vi "Tag Single Channel.vi"(0 "Data in":i16[](array[numeric])=[0, 0, 0, 0], 1 "Tag Record":bool, 2 "TagData":T1, 3 "Input Valid":bool, 4 "Tag Identifier (I16)":i16=-32768, 5 "Channel":T2(ring)) -> (7 "Single Channel Data out":i16, 8 "Output Valid":bool, 9 "Pixel Overwritten by Tag":bool)   [LabVIEW 2014]
uses:
  Frametag Data.ctl
panel:
  # "Copyright 2014 Vidrio Technologies\nScanImage 5 software is licensed under the Apache License, Version 2.0 (the \"License\"); you may not use any files contained\nwithin the ScanImage 5 release except in compliance with the License. You may obtain a copy of the License at\n http://www.apache.org/licenses/LICENSE-2.0\nUnless required by applicable law or agreed to in writing, software distributed under the License is distributed on an\n\"AS IS\" BASIS, WITHOUT WARRANTIES OR CONDITIONS OF ANY KIND, either express or implied. See the License for the\n specific language governing permissions and limitations under the License."
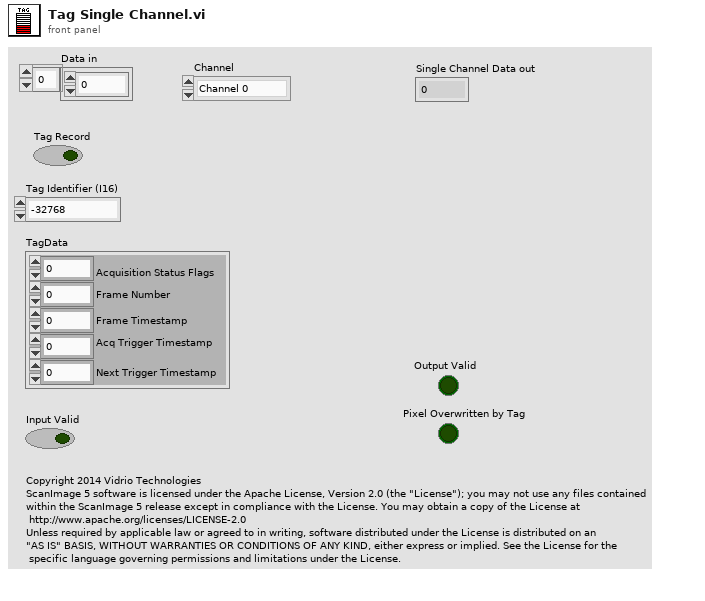
[diagram p1: front panel]
types:
  T1 = typedef "Frametag Data.ctl" = cluster{"Acquisition Status Flags":u16, "Frame Number":u32, "Frame Timestamp":u64, "Acq Trigger Timestamp":u64, "Next Trigger Timestamp":u64}
  T2 = enum8{"Channel 0", "Channel 1", "Channel 2", "Channel 3"}
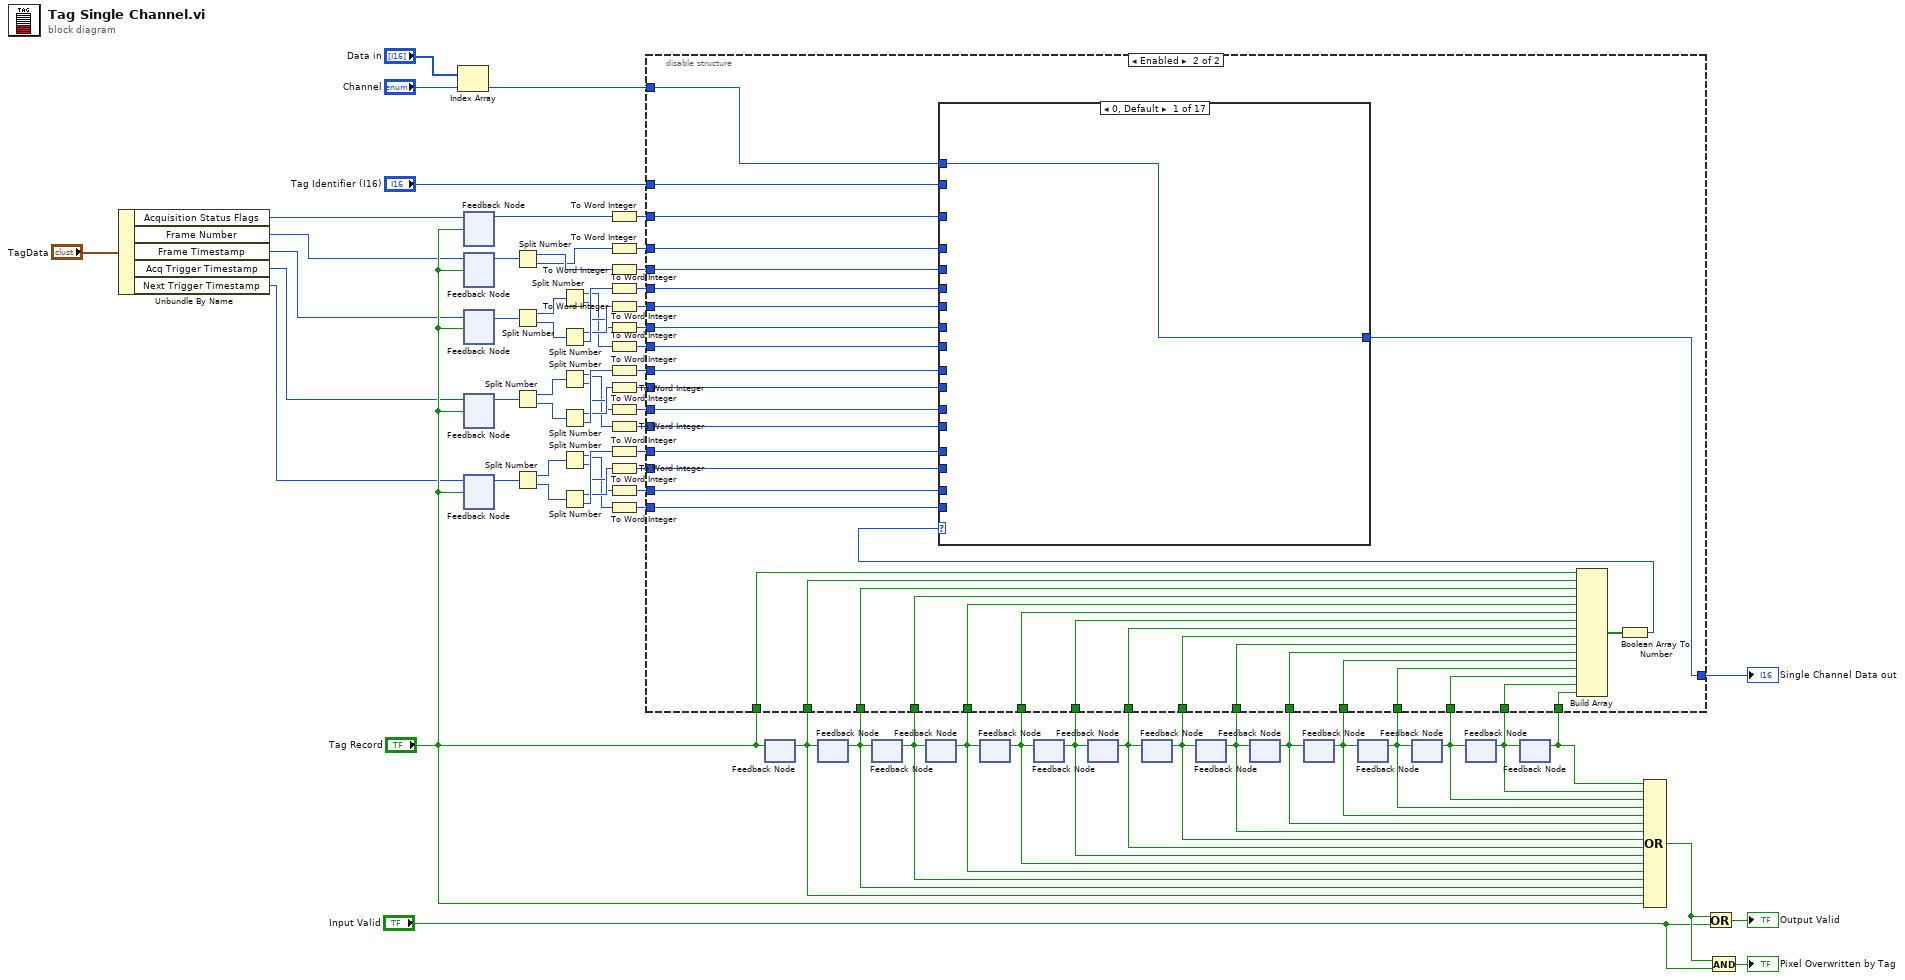
[diagram p0: block diagram]
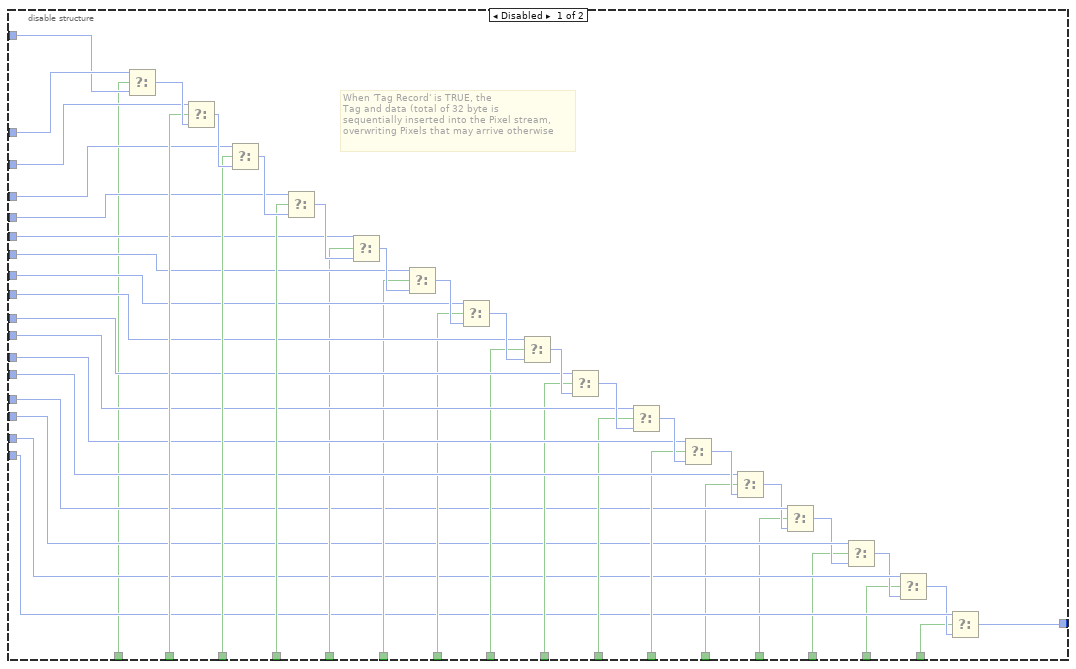
[diagram p2: hidden frame]
diagram:
  n1 = Unbundle By Name("TagData") -> ("Acquisition Status Flags"=w5:u16, "Frame Number"=w4:u32, "Frame Timestamp"=w3:u64, "Acq Trigger Timestamp"=w2:u64, "Next Trigger Timestamp"=w1:u64)
  n2 = Index Array(array="Data in", index="Channel") -> (element=w70:i16)
  n3 = feedback #1() -> (w60:u16)  [unwired: 1 in]
  n4 = feedback-in #1(w5, "Tag Record") -> ()
  n5 = feedback #2() -> (w61:u32)  [unwired: 1 in]
  n6 = feedback-in #2(w4, "Tag Record") -> ()
  n7 = feedback #3() -> (w56:u64)  [unwired: 1 in]
  n8 = feedback-in #3(w3, "Tag Record") -> ()
  n9 = feedback #4() -> (w51:u64)  [unwired: 1 in]
  n10 = feedback-in #4(w2, "Tag Record") -> ()
  n11 = feedback #5() -> (w30:u64)  [unwired: 1 in]
  n12 = feedback-in #5(w1, "Tag Record") -> ()
  n13 = Split Number(x=w61) -> (hi(x)=w20:u16, lo(x)=w19:u16)
  n14 = Split Number(x=w56) -> (hi(x)=w55:u32, lo(x)=w54:u32)
  n15 = Split Number(x=w51) -> (hi(x)=w53:u32, lo(x)=w52:u32)
  n16 = Split Number(x=w30) -> (hi(x)=w28:u32, lo(x)=w29:u32)
  n17 = Split Number(x=w55) -> (hi(x)=w15:u16, lo(x)=w16:u16)
  n18 = Split Number(x=w54) -> (hi(x)=w17:u16, lo(x)=w18:u16)
  n19 = Split Number(x=w53) -> (hi(x)=w11:u16, lo(x)=w12:u16)
  n20 = Split Number(x=w52) -> (hi(x)=w13:u16, lo(x)=w14:u16)
  n21 = Split Number(x=w28) -> (hi(x)=w7:u16, lo(x)=w8:u16)
  n22 = Split Number(x=w29) -> (hi(x)=w9:u16, lo(x)=w10:u16)
  n23 = To Word Integer(number=w60) -> (16bit integer=w59:i16)
  n24 = To Word Integer(number=w19) -> (16bit integer=w58:i16)
  n25 = To Word Integer(number=w20) -> (16bit integer=w57:i16)
  n26 = To Word Integer(number=w18) -> (16bit integer=w49:i16)
  n27 = To Word Integer(number=w17) -> (16bit integer=w48:i16)
  n28 = To Word Integer(number=w16) -> (16bit integer=w47:i16)
  n29 = To Word Integer(number=w15) -> (16bit integer=w46:i16)
  n30 = To Word Integer(number=w14) -> (16bit integer=w45:i16)
  n31 = To Word Integer(number=w13) -> (16bit integer=w44:i16)
  n32 = To Word Integer(number=w12) -> (16bit integer=w43:i16)
  n33 = To Word Integer(number=w11) -> (16bit integer=w42:i16)
  n34 = To Word Integer(number=w10) -> (16bit integer=w31:i16)
  n35 = To Word Integer(number=w9) -> (16bit integer=w32:i16)
  n36 = To Word Integer(number=w8) -> (16bit integer=w33:i16)
  n37 = To Word Integer(number=w7) -> (16bit integer=w34:i16)
  n38 = feedback #6() -> (w66:bool)  [unwired: 1 in]
  n39 = feedback-in #6("Tag Record") -> ()
  n40 = feedback #7() -> (w67:bool)  [unwired: 1 in]
  n41 = feedback-in #7(w66) -> ()
  n42 = feedback #8() -> (w50:bool)  [unwired: 1 in]
  n43 = feedback-in #8(w67) -> ()
  n44 = feedback #9() -> (w41:bool)  [unwired: 1 in]
  n45 = feedback-in #9(w50) -> ()
  n46 = feedback #10() -> (w35:bool)  [unwired: 1 in]
  n47 = feedback-in #10(w41) -> ()
  n48 = feedback #11() -> (w40:bool)  [unwired: 1 in]
  n49 = feedback-in #11(w35) -> ()
  n50 = feedback #12() -> (w39:bool)  [unwired: 1 in]
  n51 = feedback-in #12(w40) -> ()
  n52 = feedback #13() -> (w38:bool)  [unwired: 1 in]
  n53 = feedback-in #13(w39) -> ()
  n54 = feedback #14() -> (w37:bool)  [unwired: 1 in]
  n55 = feedback-in #14(w38) -> ()
  n56 = feedback #15() -> (w36:bool)  [unwired: 1 in]
  n57 = feedback-in #15(w37) -> ()
  n58 = feedback #16() -> (w26:bool)  [unwired: 1 in]
  n59 = feedback-in #16(w36) -> ()
  n60 = feedback #17() -> (w25:bool)  [unwired: 1 in]
  n61 = feedback-in #17(w26) -> ()
  n62 = feedback #18() -> (w24:bool)  [unwired: 1 in]
  n63 = feedback-in #18(w25) -> ()
  n64 = feedback #19() -> (w23:bool)  [unwired: 1 in]
  n65 = feedback-in #19(w24) -> ()
  n66 = feedback #20() -> (w22:bool)  [unwired: 1 in]
  n67 = disable-structure shown="Enabled" {
    disable-tunnel: "Tag Identifier (I16)" -> [w117 w137]
    disable-tunnel: w70 -> [w116 w138]
    disable-tunnel: w67 -> [w115 w154]
    disable-tunnel: w66 -> [w114 w155]
    disable-tunnel: w59 -> [w113 w136]
    disable-tunnel: w58 -> [w112 w135]
    disable-tunnel: w57 -> [w111 w134]
    disable-tunnel: w50 -> [w110 w153]
    disable-tunnel: w49 -> [w101 w133]
    disable-tunnel: w48 -> [w100 w132]
    disable-tunnel: w47 -> [w99 w131]
    disable-tunnel: w46 -> [w98 w130]
    disable-tunnel: w45 -> [w97 w129]
    disable-tunnel: w44 -> [w96 w128]
    disable-tunnel: w43 -> [w95 w127]
    disable-tunnel: w42 -> [w94 w126]
    disable-tunnel: w41 -> [w93 w152]
    disable-tunnel: w40 -> [w92 w150]
    disable-tunnel: w39 -> [w91 w149]
    disable-tunnel: w38 -> [w90 w148]
    disable-tunnel: w37 -> [w89 w147]
    disable-tunnel: w36 -> [w88 w146]
    disable-tunnel: w35 -> [w87 w151]
    disable-tunnel: w34 -> [w86 w123]
    disable-tunnel: w33 -> [w85 w122]
    disable-tunnel: w32 -> [w84 w124]
    disable-tunnel: w31 -> [w83 w125]
    disable-tunnel: [w79 w121] -> w27
    disable-tunnel: w26 -> [w77 w145]
    disable-tunnel: w25 -> [w76 w144]
    disable-tunnel: w24 -> [w75 w143]
    disable-tunnel: w23 -> [w74 w142]
    disable-tunnel: w22 -> [w73 w141]
    disable-tunnel: "Tag Record" -> [w72 w156]
    frame Disabled {
      # "When 'Tag Record' is TRUE, the\nTag and data (total of 32 byte is\nsequentially inserted into the Pixel stream,\noverwriting Pixels that may arrive otherwise"
      n68 = Select(t=w117, s=w72, f=w116) -> (s? t:f=w118:i16)
      n69 = Select(t=w113, s=w114, f=w118) -> (s? t:f=w119:i16)
      n70 = Select(t=w112, s=w115, f=w119) -> (s? t:f=w120:i16)
      n71 = Select(t=w111, s=w110, f=w120) -> (s? t:f=w109:i16)
      n72 = Select(t=w101, s=w93, f=w109) -> (s? t:f=w108:i16)
      n73 = Select(t=w100, s=w87, f=w108) -> (s? t:f=w107:i16)
      n74 = Select(t=w99, s=w92, f=w107) -> (s? t:f=w106:i16)
      n75 = Select(t=w98, s=w91, f=w106) -> (s? t:f=w105:i16)
      n76 = Select(t=w97, s=w90, f=w105) -> (s? t:f=w104:i16)
      n77 = Select(t=w96, s=w89, f=w104) -> (s? t:f=w103:i16)
      n78 = Select(t=w95, s=w88, f=w103) -> (s? t:f=w102:i16)
      n79 = Select(t=w94, s=w77, f=w102) -> (s? t:f=w78:i16)
      n80 = Select(t=w83, s=w76, f=w78) -> (s? t:f=w80:i16)
      n81 = Select(t=w84, s=w75, f=w80) -> (s? t:f=w81:i16)
      n82 = Select(t=w85, s=w74, f=w81) -> (s? t:f=w82:i16)
      n83 = Select(t=w86, s=w73, f=w82) -> (s? t:f=w79:i16)
    }
    frame Enabled {
      n84 = Build Array(w156, w155, w154, w153, w152, w151, w150, w149, w148, w147, w146, w145, w144, w143, w142, w141) -> (w140:bool[])
      n85 = Boolean Array To Number(Boolean array=w140) -> (number=w139:u16)
      n86 = case shown="0, Default" w139 {
        tunnel: w138 -> [w157 _ _ _ _ _ _ _ _ _ _ _ _ _ _ _ _]
        tunnel: w137 -> [_ w158 _ _ _ _ _ _ _ _ _ _ _ _ _ _ _]
        tunnel: w136 -> [_ _ w159 _ _ _ _ _ _ _ _ _ _ _ _ _ _]
        tunnel: w135 -> [_ _ _ w160 _ _ _ _ _ _ _ _ _ _ _ _ _]
        tunnel: w134 -> [_ _ _ _ w161 _ _ _ _ _ _ _ _ _ _ _ _]
        tunnel: w133 -> [_ _ _ _ _ w162 _ _ _ _ _ _ _ _ _ _ _]
        tunnel: w132 -> [_ _ _ _ _ _ w163 _ _ _ _ _ _ _ _ _ _]
        tunnel: w131 -> [_ _ _ _ _ _ _ w164 _ _ _ _ _ _ _ _ _]
        tunnel: w130 -> [_ _ _ _ _ _ _ _ w165 _ _ _ _ _ _ _ _]
        tunnel: w129 -> [_ _ _ _ _ _ _ _ _ w166 _ _ _ _ _ _ _]
        tunnel: w128 -> [_ _ _ _ _ _ _ _ _ _ w167 _ _ _ _ _ _]
        tunnel: w127 -> [_ _ _ _ _ _ _ _ _ _ _ w168 _ _ _ _ _]
        tunnel: w126 -> [_ _ _ _ _ _ _ _ _ _ _ _ w169 _ _ _ _]
        tunnel: w125 -> [_ _ _ _ _ _ _ _ _ _ _ _ _ w170 _ _ _]
        tunnel: w124 -> [_ _ _ _ _ _ _ _ _ _ _ _ _ _ w171 _ _]
        tunnel: w123 -> [_ _ _ _ _ _ _ _ _ _ _ _ _ _ _ _ w173]
        tunnel: w122 -> [_ _ _ _ _ _ _ _ _ _ _ _ _ _ _ w172 _]
        tunnel: [w157 w158 w159 w160 w161 w162 w163 w164 w165 w166 w167 w168 w169 w170 w171 w172 w173] -> w121
        frame 0, Default {
        }
        frame 1 {
        }
        frame 2 {
        }
        frame 4 {
        }
        frame 8 {
        }
        frame 16 {
        }
        frame 32 {
        }
        frame 64 {
        }
        frame 128 {
        }
        frame 256 {
        }
        frame 512 {
        }
        frame 1024 {
        }
        frame 2048 {
        }
        frame 4096 {
        }
        frame 8192 {
        }
        frame 16384 {
        }
        frame 32768 {
        }
      }
    }
  }
  "Single Channel Data out" <- w27
  n87 = feedback-in #20(w23) -> ()
  n88 = Compound Arithmetic op=OR(w22, w23, w24, w25, w26, w36, w37, w38, w39, w40, w35, w41, w50, w67, w66, "Tag Record") -> (w64:bool)
  n89 = Or(x=w64, y="Input Valid") -> (x .or. y?=→"Output Valid":bool)
  n90 = And(x=w64, y="Input Valid") -> (x .and. y?=→"Pixel Overwritten by Tag":bool)
